vi "ManipulatorPositionControl.vi"(8 "error in (no error)":errorcluster, 10 "ButtonArray":bool[](array[boolean])) -> ()   [LabVIEW 2015]
uses:
  Utilities/GeneralGlobals.vi
  Utilities/MotorPositionGlobals.vi
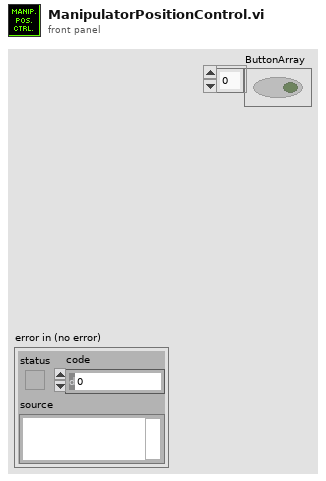
[diagram p1: front panel]
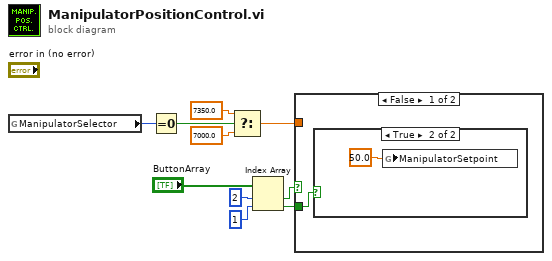
[diagram p0: block diagram]
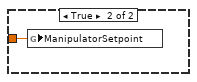
[diagram p3: hidden frame]
diagram:
  n1 = global read "GeneralGlobals.vi" "ManipulatorSelector"() -> (w6:i32)
  n2 = Equal To 0?(x=w6) -> (x = 0?=w10:bool)
  n3 = Select(t=7350.0, s=w10, f=7000.0) -> (s? t:f=w7:dbl)
  n4 = Index Array(array="ButtonArray", index #1=2 ("index"), index #2=1 ("index")) -> (element #1=w2:bool, element #2=w1:bool)
  n5 = case shown="False" w2 {
    tunnel: w7 -> [_ w13]
    tunnel: w1 -> [w11 _]
    frame False {
      n6 = case shown="True" w11 {
        frame False {
        }
        frame True {
          n7 = global write "MotorPositionGlobals.vi" "ManipulatorSetpoint"(50.0 ("ManipulatorSetpoint")) -> ()
        }
      }
    }
    frame True {
      n8 = global write "MotorPositionGlobals.vi" "ManipulatorSetpoint"(w13) -> ()
    }
  }
